vi "GetVIsToNotUpdateConnectorPanePatteronOn.vi"(0 "ClassWriterGOOP300 in":refnum<class "ClassWriterGOOP300.lvclass">, 5 "error in (no error)":errorcluster) -> (14 "ClassWriterGOOP300 out":refnum<class "ClassWriterGOOP300.lvclass">, 15 "VIsToNotUpdateConnectorPanePatteronOn":string[](array[string]), 19 "error out":errorcluster)   [LabVIEW 2020, in "ClassWriterGOOP300.lvclass"]
uses:
  ClassWriterGOOP300.lvclass
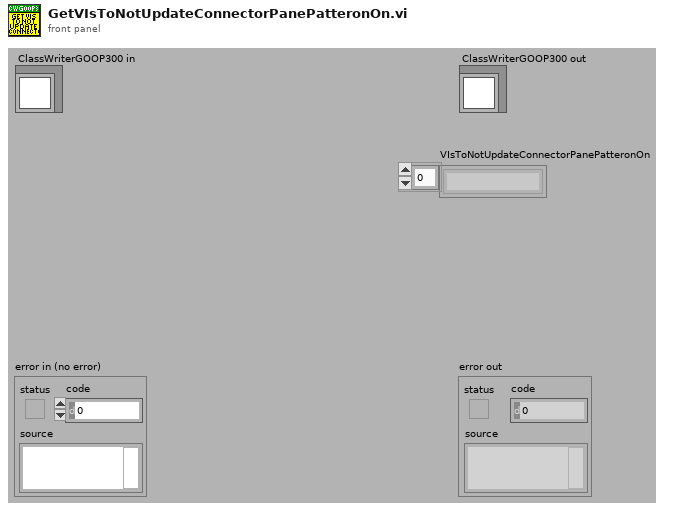
[diagram p1: front panel]
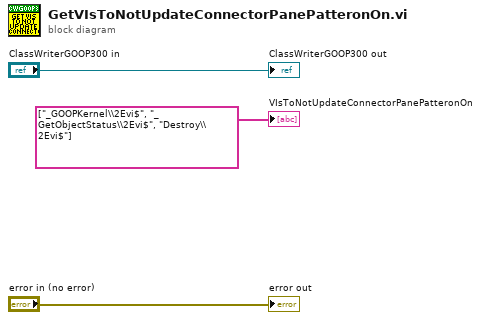
[diagram p0: block diagram]
diagram:
  "ClassWriterGOOP300 out" <- "ClassWriterGOOP300 in"
  "VIsToNotUpdateConnectorPanePatteronOn" <- string[] ["_GOOPKernel\\2Evi$", "_GetObjectStatus\\2Evi$", "Destroy\\2Evi$"] ("VIsToNotUpdateConnectorPanePatteronOn")
  "error out" <- "error in (no error)"
